vi "RichToFlatrfcontrol_SetRFDCCalibrationBypassResponse.vi"(5 "OutputClusterType":T1, 11 "InputCluster":T2) -> (3 "OutputCluster":T1)   [LabVIEW 2024, in "FlexSDR_gRPC_client.lvlib"]
uses:
  rfcontrol_SetRFDCCalibrationBypassResponse.ctl
  rfcontrol_SetRFDCCalibrationBypassResponse_Flat.ctl
  FlexSDR_gRPC_client.lvlib
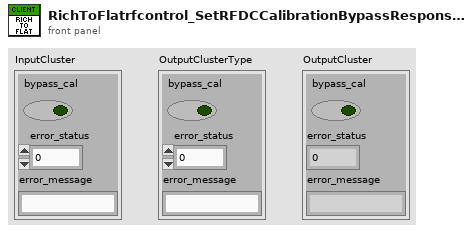
[diagram p1: front panel]
types:
  T1 = typedef "FlexSDR_gRPC_client.lvlib/rfcontrol_SetRFDCCalibrationBypassResponse_Flat.ctl" = cluster{"bypass_cal":bool, "error_status":i32, "error_message":string}
  T2 = typedef "FlexSDR_gRPC_client.lvlib/rfcontrol_SetRFDCCalibrationBypassResponse.ctl" = cluster{"bypass_cal":bool, "error_status":i32, "error_message":string}
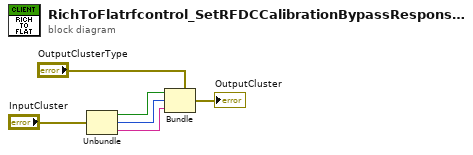
[diagram p0: block diagram]
diagram:
  n1 = Unbundle "Unbundle"("InputCluster") -> ("bypass_cal"=w3:bool, "error_status"=w2:i32, "error_message"=w1:string)
  n2 = Bundle "Bundle"(cluster="OutputClusterType", "bypass_cal"=w3, "error_status"=w2, "error_message"=w1) -> (→"OutputCluster":T1)
